vi "Constructor.vi"(8 "error in (no error)":errorcluster, 10 "Table Name (Use Member Data)":string, 11 "Table Configuration Basic DB in":refnum<class "Table Configuration Basic DB.lvclass">) -> (0 "error out":errorcluster, 3 "Table Configuration Basic DB out":refnum<class "Table Configuration Basic DB.lvclass">)   [LabVIEW 2020, in "Table.lvlib" / "Table Configuration Basic DB.lvclass"]
uses:
  Table Configuration Basic DB.lvclass
  C:/Users/User/Desktop/Raman Program/Database OOP/source/Database OOP/Table Libraries/Basic Table/Configuration/Table Configuration Class/Table Configuration.lvclass
  Table Configuration Class/Table Configuration.lvclass/Table Configuration.ctl
  Table Configuration Class/Table Configuration.lvclass
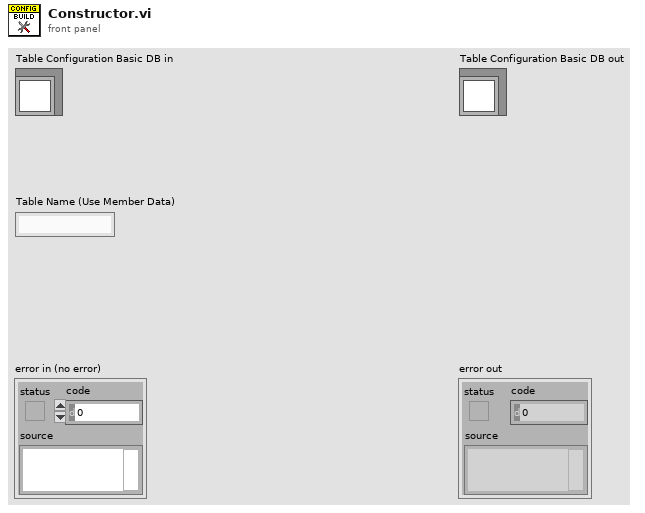
[diagram p1: front panel]
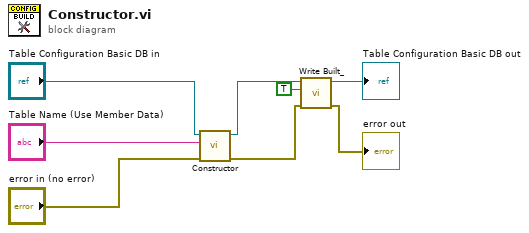
[diagram p0: block diagram]
diagram:
  n1 = call-parent "Constructor.vi"("error in (no error)"="error in (no error)", "Table Name (Use Member Data)"="Table Name (Use Member Data)", "Table Configuration in"="Table Configuration Basic DB in") -> ("error out"=w4:errorcluster, "Table Configuration out"=w6:refnum<class "Table Configuration Basic DB.lvclass">)  [unwired: 7 in]
  n2 = call "Write Built_.vi"("error in (no error)"=w4, "Built?"=TRUE, "Table Configuration in"=w6) -> ("error out"=→"error out":errorcluster, "Table Configuration out"=→"Table Configuration Basic DB out":refnum<class "Table Configuration Basic DB.lvclass">)  [unwired: 7 in]
